vi "Read UI VI Ref.vi"(8 "error in (no error)":errorcluster, 11 "Display Panel V3 in":refnum<class "Display Panel V3.lvclass">) -> (0 "error out":errorcluster, 2 "UI VI Ref":refnum<vi>, 3 "Display Panel V3 out":refnum<class "Display Panel V3.lvclass">)   [LabVIEW 2014]
uses:
  Display Panel V3.lvclass
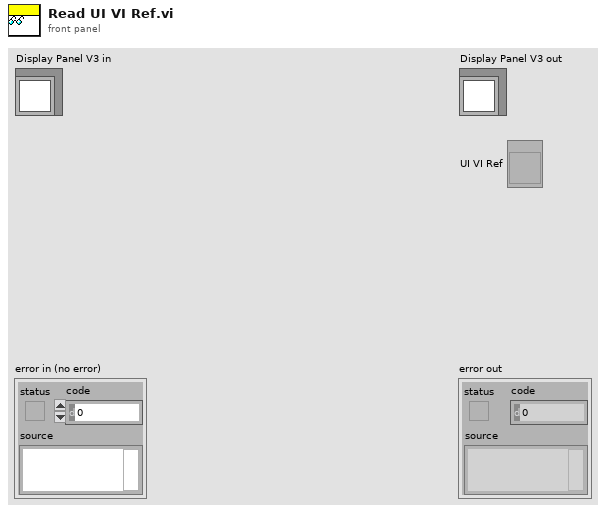
[diagram p1: front panel]
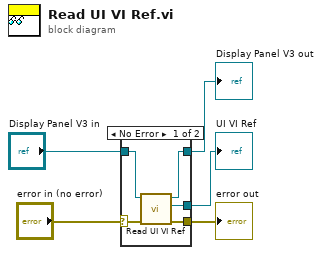
[diagram p0: block diagram]
diagram:
  n1 = case shown="No Error" "error in (no error)" {
    selector: "error in (no error)" -> [w7 w11]
    tunnel: [w6 w11] -> w4
    tunnel: [w8 w12] -> w2
    tunnel: "Display Panel V3 in" -> [w10 w12]
    tunnel: [w9 _] -> w1
    frame No Error {
      n2 = call-dynamic "Read UI VI Ref.vi"("error in (no error)"=w7, "Subpanel Inserter in"=w10) -> ("error out"=w6:errorcluster, "UI VI Ref"=w9:refnum<vi>, "Subpanel Inserter out"=w8:refnum<class "Display Panel V3.lvclass">)  [unwired: 7 in]
    }
    frame Error {
    }
  }
  "error out" <- w4
  "Display Panel V3 out" <- w2
  "UI VI Ref" <- w1
